vi "GEOM_sustitute_size.vi"(5 "detrows":i32, 7 "detcols":i32, 10 "info str":string) -> (2 "info str out":string)   [LabVIEW 2016]
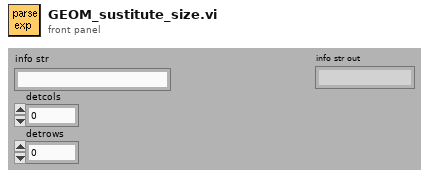
[diagram p1: front panel]
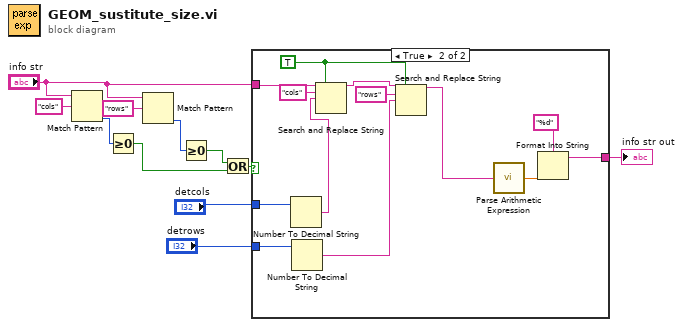
[diagram p0: block diagram]
diagram:
  n1 = Match Pattern(string="info str", regular expression="cols") -> (offset past match=w10:i32)  [unwired: 4 out]
  n2 = Greater Or Equal To 0?(x=w10) -> (x >= 0?=w7:bool)
  n3 = Match Pattern(string="info str", regular expression="rows") -> (offset past match=w9:i32)  [unwired: 4 out]
  n4 = Greater Or Equal To 0?(x=w9) -> (x >= 0?=w8:bool)
  n5 = Or(x=w8, y=w7) -> (x .or. y?=w6:bool)
  n6 = case shown="True" w6 {
    tunnel: "info str" -> [w12 w25]
    tunnel: "detcols" -> [_ w22]
    tunnel: "detrows" -> [_ w21]
    tunnel: [w12 w13] -> w2
    frame False {
    }
    frame True {
      w19 = TRUE ("replace all? (F)")
      n7 = Number To Decimal String(number=w22) -> (decimal integer string=w18:string)  [unwired: 1 out]
      n8 = Number To Decimal String(number=w21) -> (decimal integer string=w17:string)  [unwired: 1 out]
      n9 = Search and Replace String(replace all?=w19, input string=w25, search string="cols", replace string=w18) -> (result string=w20:string)  [unwired: 1 in, 6 out]
      n10 = Search and Replace String(replace all?=w19, input string=w20, search string="rows", replace string=w17) -> (result string=w16:string)  [unwired: 1 in, 6 out]
      n11 = call "Parse Arithmetic Expression.vi"("Arithmetic Expression"=w16) -> ("Result"=w15:dbl)
      n12 = Format Into String(format string="%d", w15) -> (resulting string=w13:string)  [unwired: 2 in, 1 out]
    }
  }
  "info str out" <- w2
